vi "WriteUR Core.vi"(8 "error in (no error)":errorcluster, 11 "Master CR in":refnum<class "Master CR.lvclass">) -> (0 "error out":errorcluster)   [LabVIEW 2021, in "Master CR.lvclass"]
uses:
  Master CR.lvclass
  Master CR.lvclass/Master CR.ctl
  Data Model/ICPCON ET7000 Data Model/ICPCON ET Data Model.lvclass
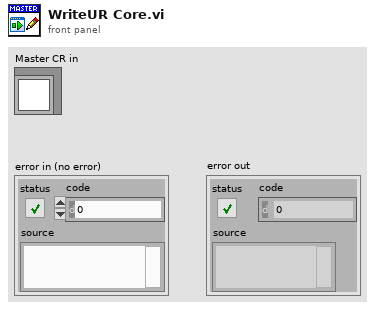
[diagram p1: front panel]
types:
  T1 = typedef "Master CR.lvclass/CR_Core_State.ctl" = enum8{"initialization", "redefine", "standby", "ping", "connect", "wait to reconnect", "wait to reset timeout", "configure", "requests", "close connection", "stop"}
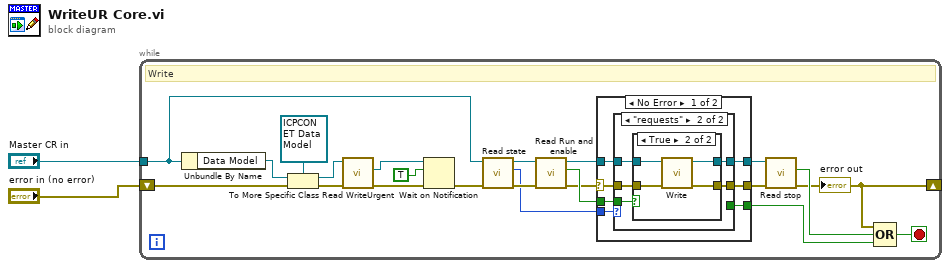
[diagram p0: block diagram]
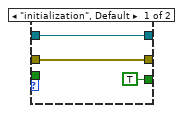
[diagram p2: hidden frame]
diagram:
  n1 = while {
    tunnel: "Master CR in" -> [w14]
    shift-right: [w16] -> _
    shift-left: "error in (no error)" -> [w9]
    stop <- w24 stop-if-true
    # "Write"
    n2 = Unbundle By Name(w14) -> ("Data Model"=w7:refnum<class "Device Data Model.lvclass">)
    n3 = To More Specific Class(target class=refnum<class "ICPCON ET Data Model.lvclass"> refnum ("Device Data Model"), reference=w7, error in=w9) -> (specific class reference=w5:refnum<class "ICPCON ET Data Model.lvclass">, error out=w8:errorcluster)
    n4 = call "Read WriteUrgent.vi"("error in (no error)"=w8, "ICPCON ET Data Model in"=w5) -> ("error out"=w4:errorcluster, "WriteUrgent"=w3:refnum<notifier>)  [unwired: 7 in, 1 out]
    n5 = Wait on Notification(notifier=w3, ignore previous (F)=TRUE, error in (no error)=w4) -> (error out=w10:errorcluster)  [unwired: 1 in, 3 out]
    n6 = call "Read state.vi"("error in (no error)"=w10, "Master CR in"=w14) -> ("error out"=w20:errorcluster, "state"=w19:T1, "Master CR out"=w13:refnum<class "Master CR.lvclass">)  [unwired: 7 in]
    n7 = call "Read Run and enable.vi"("error in (no error)"=w20, "Master CR in"=w13) -> ("error out"=w11:errorcluster, "Enable and Run"=w18:bool, "Master CR out"=w12:refnum<class "Master CR.lvclass">)  [unwired: 7 in]
    n8 = case shown="No Error" w11 {
      selector: w11 -> [w27 w46]
      tunnel: w12 -> [w26 w47]
      tunnel: [w31 w46] -> w22
      tunnel: [w30 w47] -> w21
      tunnel: w19 -> [w29 _]
      tunnel: w18 -> [w28 _]
      tunnel: [w25 _] -> w15
      frame No Error {
        n9 = case shown="\"requests\"" w29 {
          tunnel: w28 -> [_ w39]
          tunnel: w26 -> [w33 w38]
          tunnel: w27 -> [w34 w37]
          tunnel: [w34 w36] -> w31
          tunnel: [w33 w35] -> w30
          tunnel: [TRUE ("ignore previous (F)") _] -> w25
          frame "initialization", Default {
          }
          frame "requests" {
            n10 = case shown="True" w39 {
              tunnel: w38 -> [w40 w44]
              tunnel: w37 -> [w41 w45]
              tunnel: [w41 w43] -> w36
              tunnel: [w40 w42] -> w35
              frame False {
              }
              frame True {
                n11 = call-dynamic "Write.vi"("error in (no error)"=w45, "MB_TCP in"=w44) -> ("error out"=w43:errorcluster, "MB_TCP out"=w42:refnum<class "Master CR.lvclass">)  [unwired: 8 in]
              }
            }
          }
        }
      }
      frame Error {
      }
    }
    n12 = call "Read stop.vi"("error in (no error)"=w22, "Master CR in"=w21) -> ("error out"=w16:errorcluster, "Stop"=w17:bool)  [unwired: 7 in, 1 out]
    "error out" <- w16
    n13 = Compound Arithmetic op=OR(w16, w17, w15) -> (w24:bool)
  }
